vi "Newmark-InitSpeed.vi"(0 "Table VRN":refnum<visa-resource-name>="COM9", 2 "StageTags":string[](array[string]), 7 "Bool Refnum":refnum<vi>, 9 "Vitesse Foyer":dbl, 11 "Error IN":errorcluster, 12 "Vitesse Lente":dbl, 13 "Vitesse Rapide":dbl, 14 "Accélération":dbl) -> (4 "Table VRN OUT":refnum<visa-resource-name>="COM9", 8 "Erreur?":bool, 15 "Error OUT":errorcluster)   [LabVIEW 2011]
panel:
  # "[mm/sec]"
  # "[mm/sec]"
  # "[mm/sec/sec]"
  # "Il faudra probablement vérifier l'ordre dans lequel envoyer les\nvitesse pour respecter l'ordre croissant :\n\nFast en premier, mais si fast en plus petit que la vitesse actuellement\nminimale, on a un problème et on recevra un '#'\n\nNormalement, cela a été réglé ..."
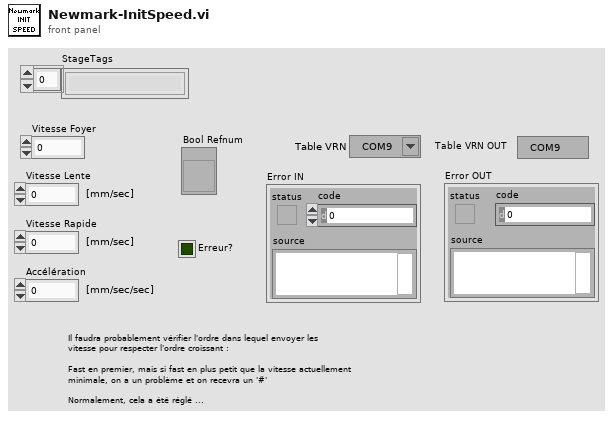
[diagram p1: front panel]
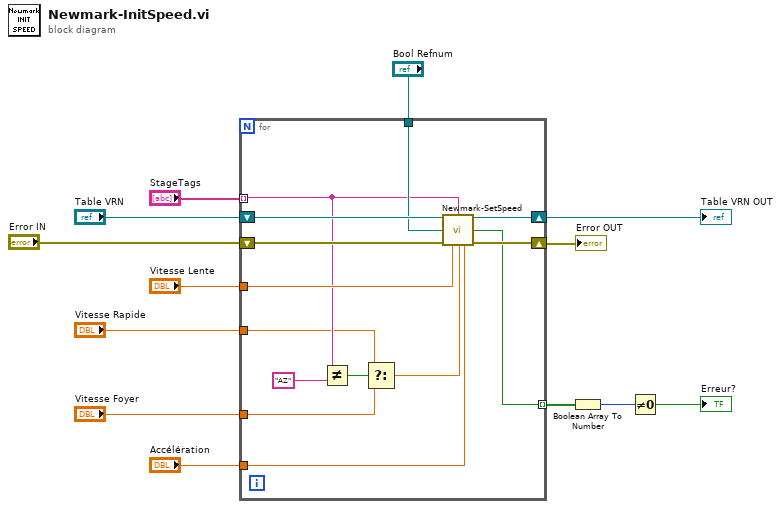
[diagram p0: block diagram]
diagram:
  n1 = for {
    tunnel: "StageTags" -> [w18] mode=indexing
    tunnel: "Vitesse Lente" -> [w27]
    tunnel: "Accélération" -> [w26]
    tunnel: "Bool Refnum" -> [w23]
    shift-right: [w22] -> w7
    shift-left: "Table VRN" -> [w25]
    shift-right: [w21] -> w6
    shift-left: "Error IN" -> [w24]
    tunnel: [w20] -> w5 mode=indexing
    tunnel: "Vitesse Rapide" -> [w16]
    tunnel: "Vitesse Foyer" -> [w15]
    n2 = Not Equal?(x=w18, y="AZ") -> (x != y?=w17:bool)
    n3 = Select(t=w16, s=w17, f=w15) -> (s? t:f=w14:dbl)
    n4 = call "Newmark-SetSpeed.vi"("Table VRN"=w25, "StageTAG"=w18, "Bool Refnum"=w23, "Error IN"=w24, "Vitesse Lente"=w27, "Vitesse Rapide"=w14, "Accélération"=w26) -> ("Table VRN OUT"=w22:refnum<visa-resource-name>, "Erreur?"=w20:bool, "Error OUT"=w21:errorcluster)  [unwired: 6 in]
  }
  "Error OUT" <- w6
  "Table VRN OUT" <- w7
  n5 = Boolean Array To Number(Boolean array=w5) -> (number=w4:u32)
  n6 = Not Equal To 0?(x=w4) -> (x != 0?=→"Erreur?":bool)
